vi "RP Scale.vi"(10 "Signal bits":i32=14, 11 "Range":dbl=1.0 format="%#_6eV") -> (3 "Scale":dbl)   [LabVIEW 2015]
panel:
  out "x << y":i32
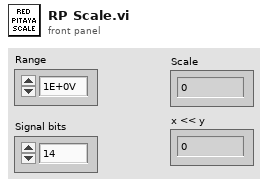
[diagram p1: front panel]
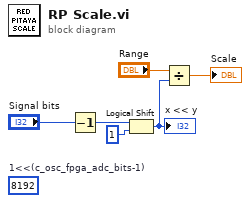
[diagram p0: block diagram]
diagram:
  (unwired) 8192  # 1<<(c_osc_fpga_adc_bits-1)
  n1 = Decrement(x="Signal bits") -> (x-1=w6:i32)
  n2 = Logical Shift(y=w6, x=1) -> (x << y=w3:i32)
  "x << y" <- w3
  n3 = Divide(x="Range", y=w3) -> (x/y=→"Scale":dbl)
